vi "InsertWaitIntoError.vi"(2 "error in (no error)":errorcluster, 3 "Wait (msecs)":dbl) -> (0 "error out":errorcluster)   [LabVIEW 2012]
doc: "Insert a delay, in msecs, into an error stream."
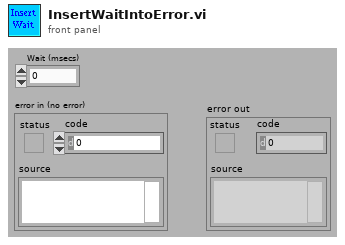
[diagram p1: front panel]
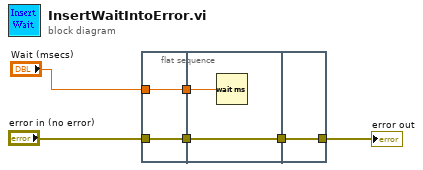
[diagram p0: block diagram]
diagram:
  n1 = flat-sequence {
    tunnel: "Wait (msecs)" -> [w8]
    tunnel: [w8] -> w5
    tunnel: [w7] -> w4
    tunnel: "error in (no error)" -> [w7]
    tunnel: w5 -> [w10]
    tunnel: w4 -> [w9]
    tunnel: [w9] -> w2
    tunnel: w2 -> [w11]
    tunnel: [w11] -> w1
    frame #0 {
    }
    frame #1 {
      n2 = Wait (ms)(milliseconds to wait=w10) -> ()  [unwired: 1 out]
    }
    frame #2 {
    }
  }
  "error out" <- w1
